vi "New.vi"(5 "Center on Canvas":bool, 7 "Origin at Center":bool, 8 "error in (no error)":errorcluster, 11 "3x3 Matrix (Identity)":T1=[[1.0, 0.0, 0.0], [0.0, 1.0, 0.0], [0.0, 0.0, 1.0]]) -> (0 "error out":errorcluster, 3 "Static Image Transform out":refnum<class "Static Image Transform.lvclass">)   [LabVIEW 2023, in "Font Glyph Drawer Interface.lvlib" / "Static Image Transform.lvclass"]
uses:
  Static Image Transform.lvclass
  <vilib>/Analysis/Matrix/Datatypes/RealMatrix.ctl
  Static Image Transform.lvclass/Static Image Transform.ctl
  <vilib>/Analysis/Matrix/NI_Matrix.lvlib
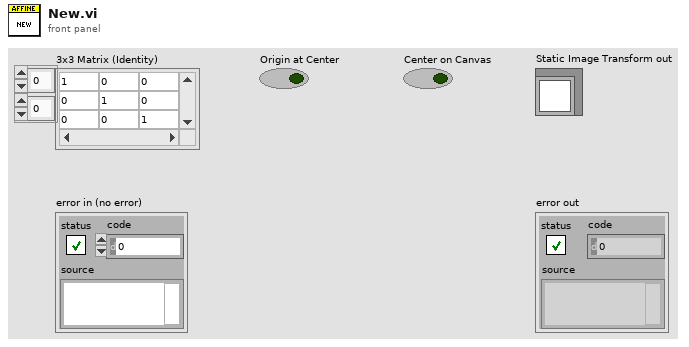
[diagram p1: front panel]
types:
  T1 = typedef "NI_Matrix.lvlib/RealMatrix.ctl" = dbl[][]
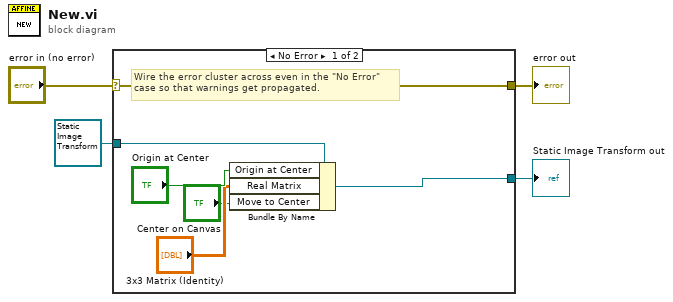
[diagram p0: block diagram]
diagram:
  n1 = case shown="No Error" "error in (no error)" {
    selector: "error in (no error)" -> [w9 w12]
    tunnel: [w9 w12] -> w3
    tunnel: [w8 w11] -> w1
    tunnel: refnum<class "Static Image Transform.lvclass"> refnum ("Static Image Transform in") -> [w10 w11]
    frame No Error {
      # "Wire the error cluster across even in the \"No Error\"\ncase so that warnings get propagated."
      n2 = Bundle By Name(cluster=w10, "Origin at Center"="Origin at Center", "Real Matrix"="3x3 Matrix (Identity)", "Move to Center"="Center on Canvas") -> (w8:refnum<class "Static Image Transform.lvclass">)
    }
    frame Error {
    }
  }
  "error out" <- w3
  "Static Image Transform out" <- w1
